vi "Problema2_4.vi"() -> ()   [LabVIEW 2020]
panel:
  out "Resultado":string
  in  "division":bool
  in  "multiplicacion":bool
  in  "resta":bool
  in  "suma":bool
  in  "Segundo valor":dbl
  in  "Primer valor":dbl
  # "Datos."
  # "Operacion a realizar."
  # "El codigo realiza las diferentes operaciones basicas, el usuario debe ingresar los balores para sus operaciones y escoger la operacion a realizar"
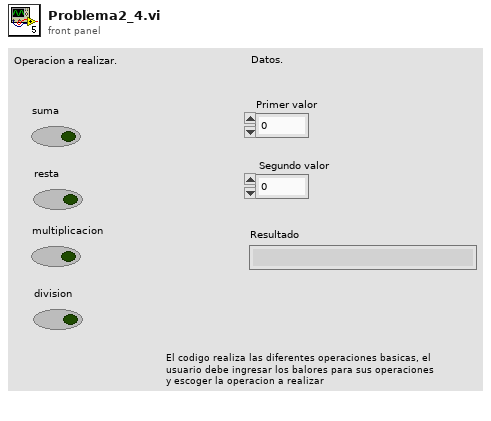
[diagram p1: front panel]
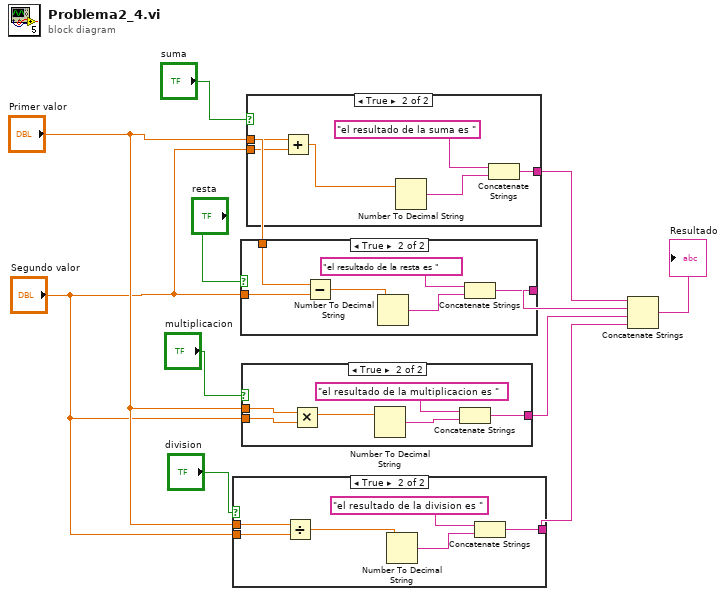
[diagram p0: block diagram]
diagram:
  n1 = case shown="True" "division" {
    tunnel: "Primer valor" -> [_ w17]
    tunnel: "Segundo valor" -> [_ w16]
    tunnel: [_ w12] -> w2
    frame False {
    }
    frame True {
      n2 = Divide(x=w17, y=w16) -> (x/y=w13:dbl)
      n3 = Number To Decimal String(number=w13) -> (decimal integer string=w14:string)  [unwired: 1 in]
      n4 = Concatenate Strings("el resultado de la division es ", w14) -> (w12:string)
    }
  }
  n5 = case shown="True" "resta" {
    tunnel: "Primer valor" -> [_ w23]
    tunnel: "Segundo valor" -> [_ w22]
    tunnel: [_ w18] -> w4
    frame False {
    }
    frame True {
      n6 = Subtract(x=w23, y=w22) -> (x-y=w19:dbl)
      n7 = Number To Decimal String(number=w19) -> (decimal integer string=w20:string)  [unwired: 1 in]
      n8 = Concatenate Strings("el resultado de la resta es ", w20) -> (w18:string)
    }
  }
  n9 = case shown="True" "multiplicacion" {
    tunnel: "Primer valor" -> [_ w29]
    tunnel: "Segundo valor" -> [_ w28]
    tunnel: [_ w24] -> w3
    frame False {
    }
    frame True {
      n10 = Multiply(x=w29, y=w28) -> (x*y=w25:dbl)
      n11 = Number To Decimal String(number=w25) -> (decimal integer string=w26:string)  [unwired: 1 in]
      n12 = Concatenate Strings("el resultado de la multiplicacion es ", w26) -> (w24:string)
    }
  }
  n13 = case shown="True" "suma" {
    tunnel: "Primer valor" -> [_ w35]
    tunnel: "Segundo valor" -> [_ w34]
    tunnel: [_ w30] -> w5
    frame False {
    }
    frame True {
      n14 = Add(x=w35, y=w34) -> (x+y=w31:dbl)
      n15 = Number To Decimal String(number=w31) -> (decimal integer string=w32:string)  [unwired: 1 in]
      n16 = Concatenate Strings("el resultado de la suma es ", w32) -> (w30:string)
    }
  }
  n17 = Concatenate Strings(w5, w4, w3, w2) -> (→"Resultado":string)
